vi "Save as HDF5.vi"(10 "Waveform 2":waveform(dbl), 11 "path":path=path "test.h5") -> ()   [LabVIEW 2017]
uses:
  <vilib>/addons/h5labview2/file/H5Fmode.ctl
  <vilib>/addons/h5labview2/base/lib_path.vi
  <vilib>/addons/h5labview2/base/H5Equery.vi
  <vilib>/addons/h5labview2/dataset/H5Dwrite.llb/H5Dwrite.xnode
  <vilib>/addons/h5labview2/dataset/H5Dread.llb/H5Dread.xnode
  <vilib>/addons/h5labview2/file/H5F.lvlib
panel:
  out "Waveform":waveform(dbl)(graph)
  out "size(s)":i32
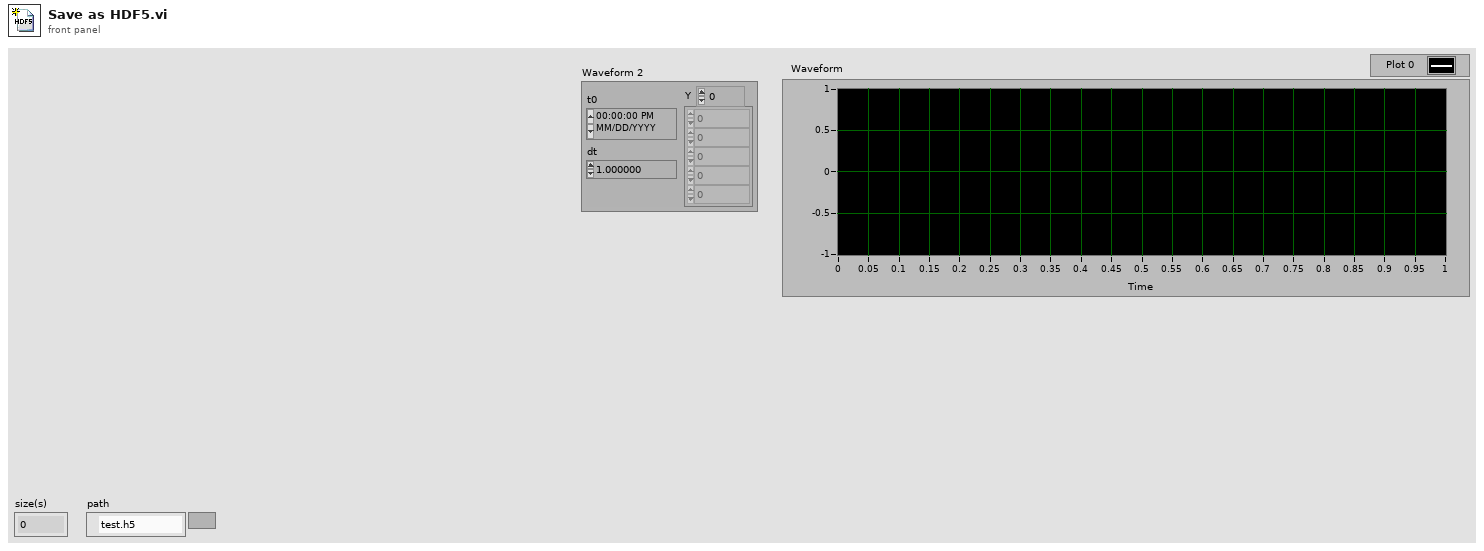
[diagram p1: front panel]
types:
  T1 = typedef "H5F.lvlib/H5Fmode.ctl" = enum16{"read-only", "read-write", "overwrite", "create new", "open or create"}
  T2 = typedef "hid_t.ctl" = i32
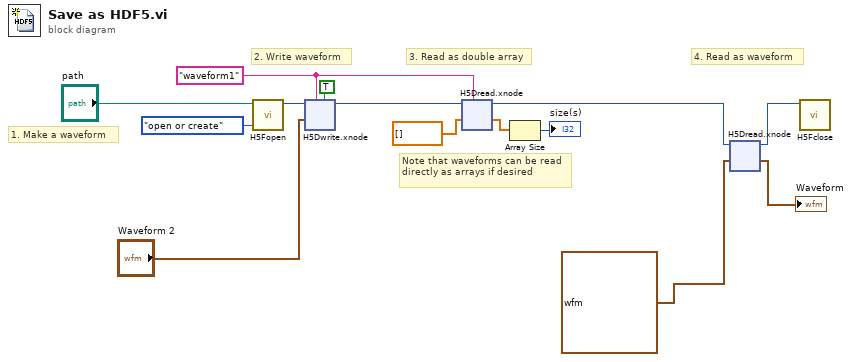
[diagram p0: block diagram]
diagram:
  w9 = "waveform1" ("dataset name")
  # "Note that waveforms can be read directly as arrays if desired"
  # "4. Read as waveform"
  # "3. Read as double array"
  # "2. Write waveform"
  # "1. Make a waveform"
  n1 = call <vilib>:"H5Fopen.vi"("mode (read-only)"=H5Fmode."open or create", "path"="path") -> ("ref out"=w14:T2)  [unwired: 8 in, 1 out]
  n2 = xnode "H5Dwrite.xnode"("replace? (F)"=TRUE, "dataset name"=w9, "data"="Waveform 2", "ref in"=w14) -> ("ref out"=w11:i32)  [unwired: 3 in, 2 out]
  n3 = xnode "H5Dread.xnode"("dataset name (this)"=w9, "default"=dbl[] [], "ref in"=w11) -> ("data"=w8:dbl[], "ref out"=w5:i32)  [unwired: 3 in, 2 out]
  n4 = Array Size(array=w8) -> (size(s)=→"size(s)":i32)
  n5 = xnode "H5Dread.xnode"("default"=waveform(dbl) {"t0"=timestamp(0 s since 1904-01-01), "dt"=1.0, "Y"=[]} ("output waveform"), "ref in"=w5) -> ("data"=→"Waveform":waveform(dbl), "ref out"=w4:i32)  [unwired: 4 in, 2 out]
  n6 = call <vilib>:"H5Fclose.vi"("ref"=w4) -> ()  [unwired: 10 in, 1 out]
